vi "Configure.vi"(8 "error in (no error)":errorcluster, 10 "Msg in":T1, 11 "FakePressureController in":refnum<class "Ztec4611.lvclass">) -> (0 "error out":errorcluster, 1 "new command":string, 2 "Msg out":T1, 3 "FakePressureController out":refnum<class "Ztec4611.lvclass">)   [LabVIEW 2011, in "Ztec4611.lvclass"]
uses:
  Ztec4611.lvclass
  DriverMsg.ctl
  Ztec4611.lvclass/Ztec4611.ctl
  impedance_Enum_TypDEf.ctl
  OnOffTypeDef.ctl
  coupling_Enum_TypDef.ctl
  TriggerSource_TypDef.ctl
  positive_negatice2_typDef.ctl
  mode_TypDef.ctl
  BaseDriver/BaseDriver.lvclass
panel:
  out "Command":string
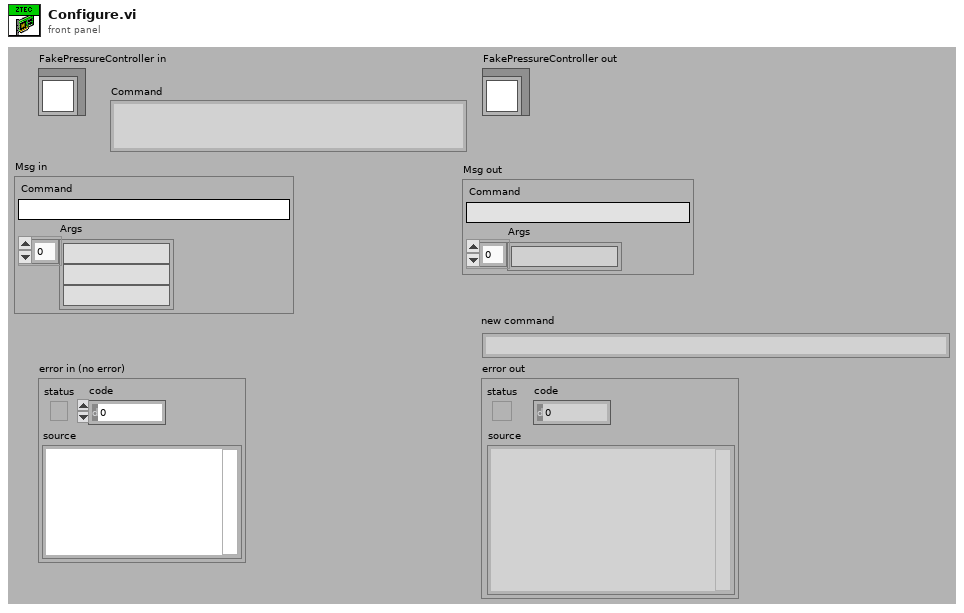
[diagram p1: front panel]
types:
  T1 = typedef "DriverMsg.ctl" = cluster{"Command":string, "Args":string[]}
  T2 = typedef "impedance_Enum_TypDEf.ctl" = enum16{"1 mega ohm", "<NA>", "50 ohms"}
  T3 = typedef "OnOffTypeDef.ctl" = enum16{"off", "on"}
  T4 = typedef "coupling_Enum_TypDef.ctl" = enum16{"AC", "DC", "Ground"}
  T5 = typedef "TriggerSource_TypDef.ctl" = enum16{"Channel 0", "Channel 1", "External TRIG"}
  T6 = typedef "positive_negatice2_typDef.ctl" = enum16{"Positive", "Negative"}
  T7 = typedef "mode_TypDef.ctl" = enum32{"Immediate", "Analog Edge", "Analog Window", "Analog Hysteresis", "Video", "Digital Edge"}
  T8 = typedef "Ztec4611.lvclass/settings_TypDef.ctl" = cluster{"resourcename":string, "timeout":T9, "LocalSavingPath":path, "Save":T3, "probeattenuation":cluster{"Channel0":T9, "Channel1":T9, "Channel2":T9, "Channel3":T9, "Channel4":T9, "Channel5":T9, "Channel6":T9, "Channel7":T9}, "channelenabled":T10, "coupling":cluster{"Channel0":T4, "Channel1":T4, "Channel2":T4, "Channel3":T4, "Channel4":T4, "Channel5":T4, "Channel6":T4, "Channel7":T4}, "impedance":cluster{"Channel0":T2, "Channel1":T2, "Channel2":T2, "Channel3":T2, "Channel4":T2, "Channel5":T2, "Channel6":T2, "Channel7":T2}, "Trigger":cluster{"Slope":T6, "AnalogSource":T5, "Low Level":dbl, "Delay":dbl, "Mode":T7}, "Horizontal":T11, "Names":cluster{"Channel0":string, "Channel1":string, "Channel2":string, "Channel3":string, "Channel4":string, "Channel5":string, "Channel6":string, "Channel7":string}, "verticalrange":cluster{"Channel0":T9, "Channel1":T9, "Channel2":T9, "Channel3":T9, "Channel4":T9, "Channel5":T9, "Channel6":T9, "Channel7":T9}, "offset":cluster{"Channel0":T9, "Channel1":T9, "Channel2":T9, "Channel3":T9, "Channel4":T9, "Channel5":T9, "Channel6":T9, "Channel7":T9}, "Number of channels":dbl, "Method":T12, "LinkedChannel":T14}
  T9 = typedef "numericVariable_TypeDef.ctl" = cluster{"Value":dbl, "Min":dbl, "Max":dbl, "StepSize":dbl, "Tolerance":dbl, "valueactual":dbl}
  T10 = typedef "channelenabled_TypDef.ctl" = cluster{"Channel0":T3, "Channel1":T3, "Channel2":T3, "Channel3":T3, "Channel4":T3, "Channel5":T3, "Channel6":T3, "Channel7":T3}
  T11 = typedef "horizontal_TypDef.ctl" = cluster{"min sample rate":dbl, "min record length":i32, "actual record length":i32, "actual sample rate":dbl, "Enforce Realtime":T3}
  T12 = typedef "methodCluster_TypDEf.ctl" = cluster{"Analysis1":T13, "Analysis2":T13, "Analysis3":T13, "Analysis4":T13, "Analysis5":T13, "Analysis6":T13, "Analysis7":T13, "Analysis8":T13, "Analysis9":T13, "Analysis10":T13}
  T13 = typedef "method_TypDef.ctl" = enum16{"n/a", "max", "min", "energy"}
  T14 = typedef "LinkedChannelsCluster_TypDef.ctl" = cluster{"Analysis1":T15, "Analysis2":T15, "Analysis3":T15, "Analysis4":T15, "Analysis5":T15, "Analysis6":T15, "Analysis7":T15, "Analysis8":T15, "Analysis9":T15, "Analysis10":T15}
  T15 = typedef "channels_TypDef.ctl" = enum16{"Channel0", "Channel1", "Channel2", "Channel3", "Channel4", "Channel5", "Channel6", "Channel7", "n/a"}
  T16 = cluster{"Channel0":T2, "Channel1":T2, "Channel2":T2, "Channel3":T2, "Channel4":T2, "Channel5":T2, "Channel6":T2, "Channel7":T2}
  T17 = cluster{"Channel0":T4, "Channel1":T4, "Channel2":T4, "Channel3":T4, "Channel4":T4, "Channel5":T4, "Channel6":T4, "Channel7":T4}
  T18 = cluster{"Channel0":T9, "Channel1":T9, "Channel2":T9, "Channel3":T9, "Channel4":T9, "Channel5":T9, "Channel6":T9, "Channel7":T9}
  T19 = cluster{"Channel0":string, "Channel1":string, "Channel2":string, "Channel3":string, "Channel4":string, "Channel5":string, "Channel6":string, "Channel7":string}
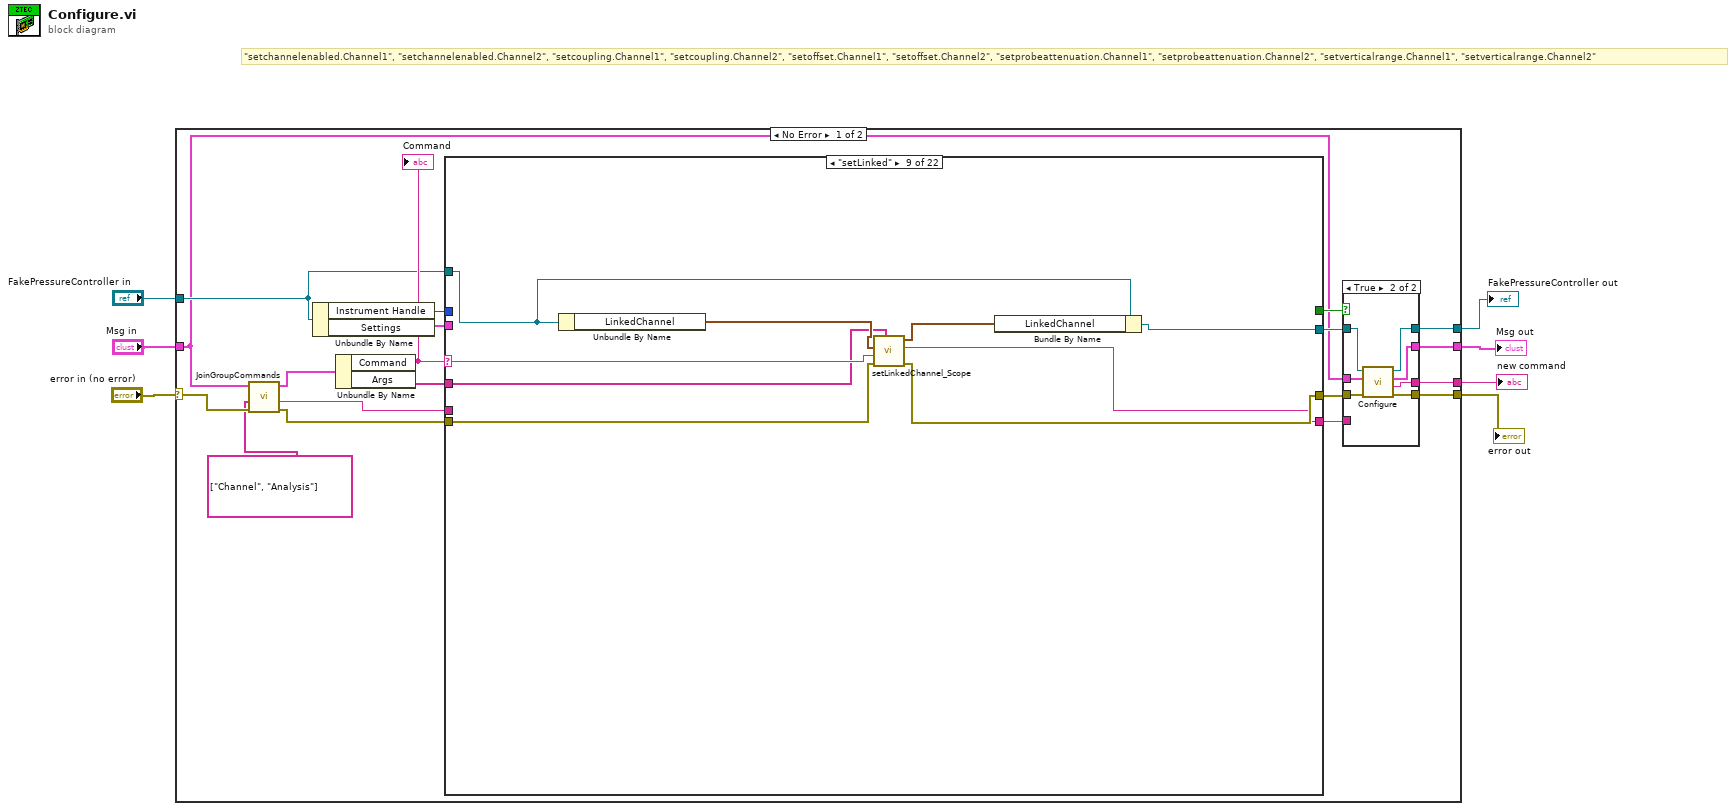
[diagram p0: block diagram]
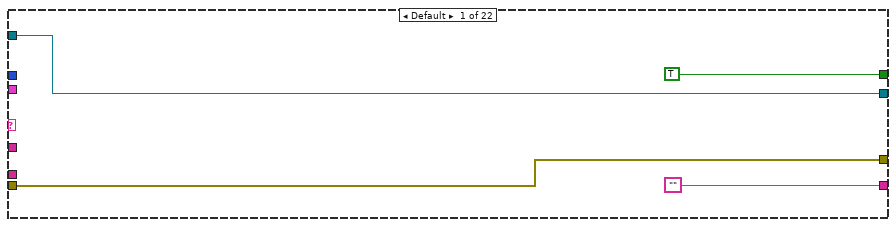
[diagram p3: hidden frame]
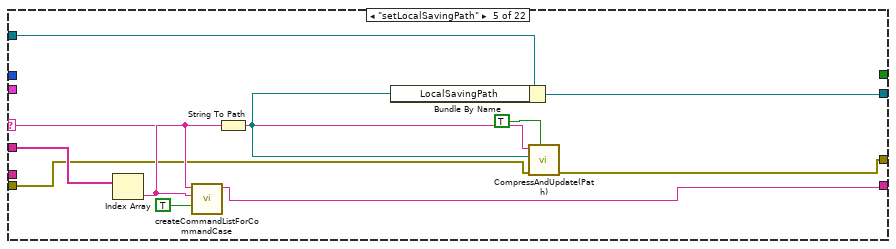
[diagram p7: hidden frame]
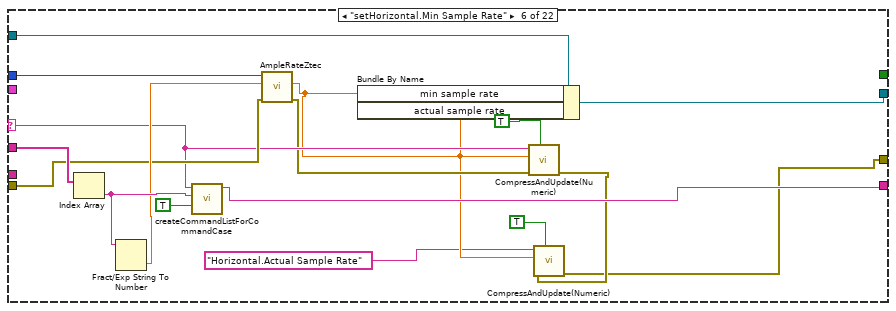
[diagram p8: hidden frame]
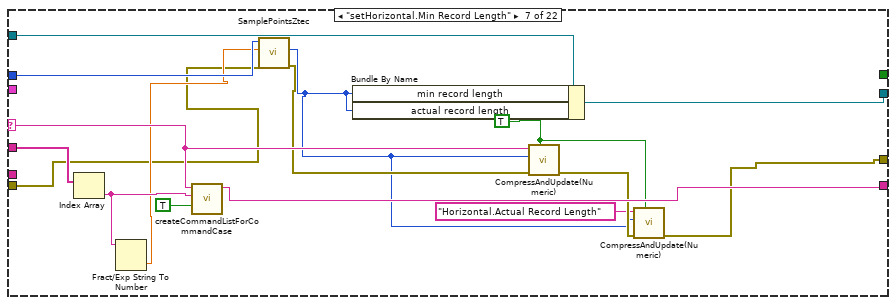
[diagram p9: hidden frame]
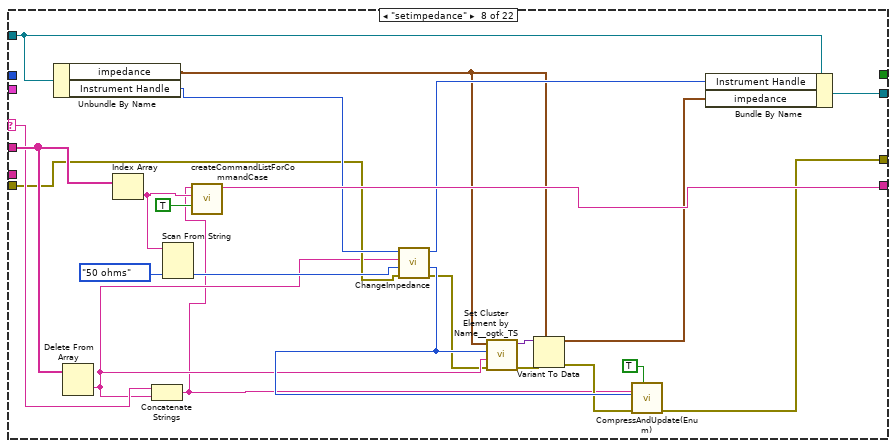
[diagram p10: hidden frame]
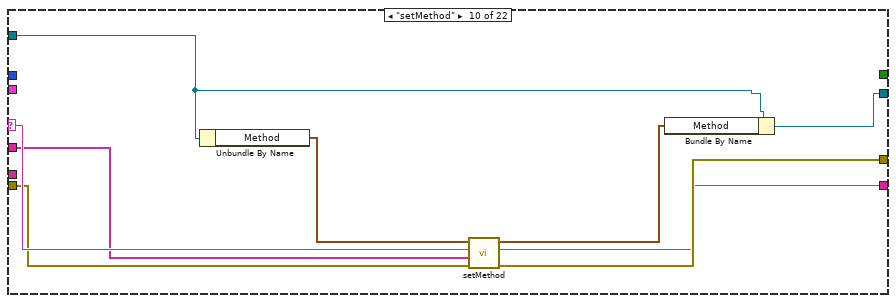
[diagram p11: hidden frame]
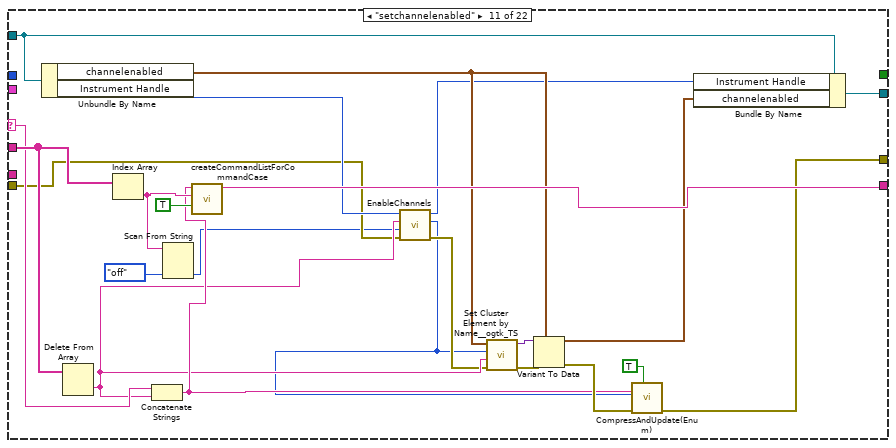
[diagram p12: hidden frame]
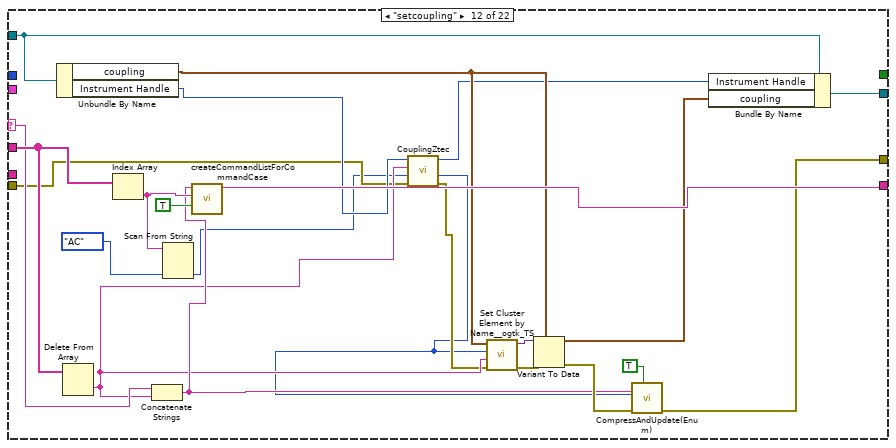
[diagram p13: hidden frame]
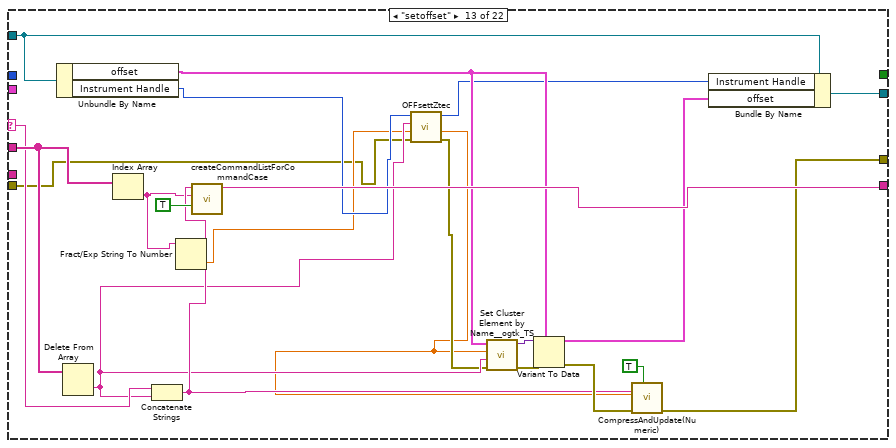
[diagram p14: hidden frame]
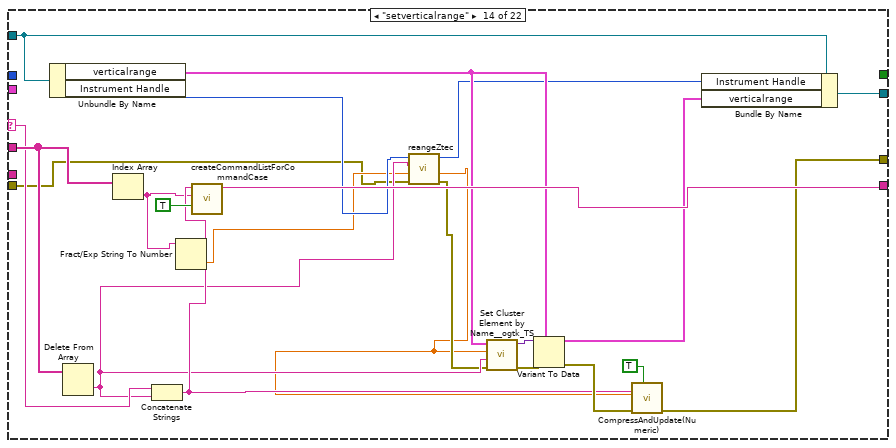
[diagram p15: hidden frame]
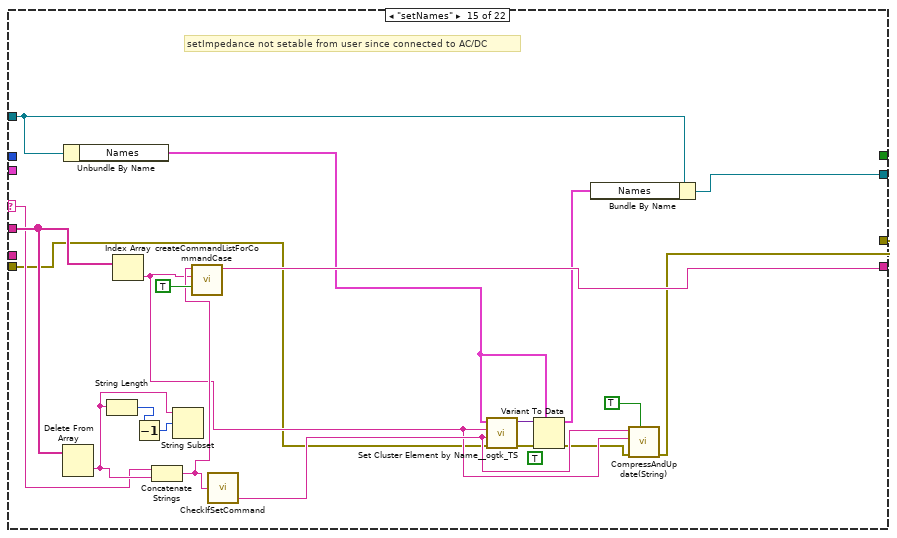
[diagram p16: hidden frame]
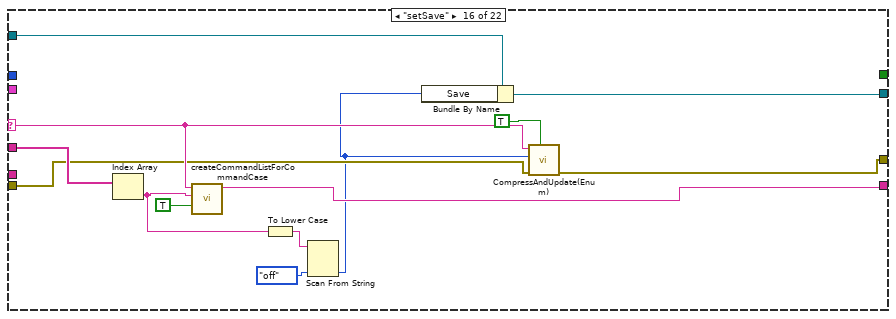
[diagram p17: hidden frame]
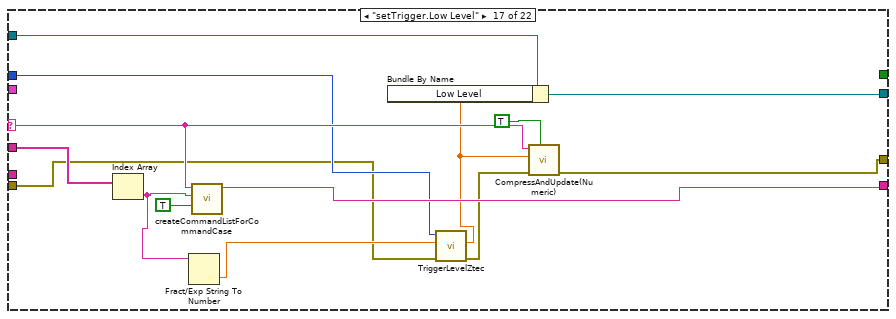
[diagram p18: hidden frame]
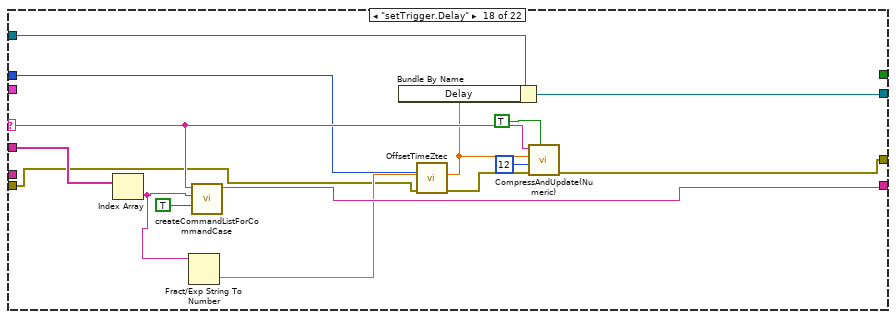
[diagram p19: hidden frame]
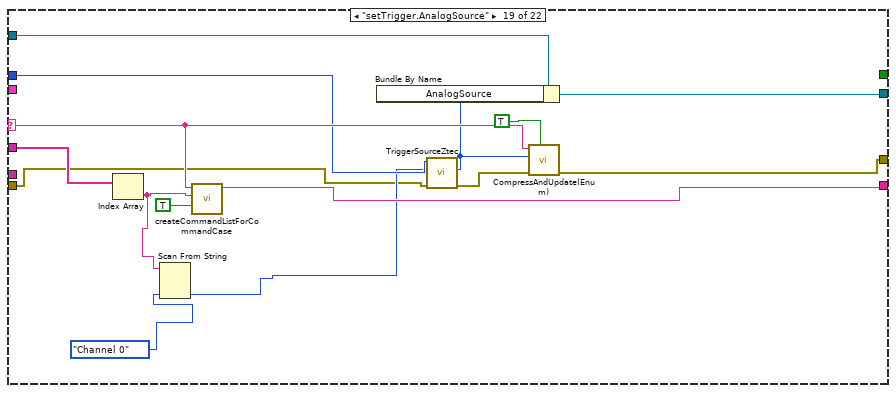
[diagram p20: hidden frame]
diagram:
  # "\"setchannelenabled.Channel1\", \"setchannelenabled.Channel2\", \"setcoupling.Channel1\", \"setcoupling.Channel2\", \"setoffset.Channel1\", \"setoffset.Channel2\", \"setprobeattenuation.Channel1\", \"setprobeattenuation.Channel2\", \"setverticalrange.Channel1\", \"setverticalrange.Channel2\""
  n1 = case shown="No Error" "error in (no error)" {
    selector: "error in (no error)" -> [w13 w356]
    tunnel: "FakePressureController in" -> [w17 w354]
    tunnel: [w25 w354] -> w4
    tunnel: [w23 w356] -> w1
    tunnel: "Msg in" -> [w10 w355]
    tunnel: [w21 w355] -> w3
    tunnel: [w19 _] -> w2
    frame No Error {
      n2 = call "JoinGroupCommands.vi"("error in (no error)"=w13, "Seperator"=string[] ["Channel", "Analysis"], "Msg in"=w10) -> ("error out"=w12:errorcluster, "Seperator out"=w9:string, "Msg out"=w11:T1)  [unwired: 6 in]
      n3 = Unbundle By Name(w17) -> ("Instrument Handle"=w16:i32, "Settings"=w15:T8)
      n4 = Unbundle By Name(w11) -> ("Command"=w18:string, "Args"=w14:string[])
      "Command" <- w18
      n5 = case shown="\"setLinked\"" w18 {
        selector: w18 -> [_ _ _ _ w53 w65 w85 w104 w116 w128 w146 w169 w192 w214 w231 w251 w265 w280 w295 w310 w338 w349]
        tunnel: w12 -> [w40 w43 w45 w46 w50 w66 w82 w99 w119 w126 w136 w161 w181 w203 w225 w249 w257 w273 w287 w304 w333 w347]
        tunnel: w14 -> [_ _ _ _ w56 w73 w89 w108 w115 w127 w150 w173 w196 w218 w236 w253 w267 w282 w297 w312 w340 w351]
        tunnel: w17 -> [w41 w42 w44 w47 w58 w75 w91 w111 w121 w130 w152 w175 w197 w219 w239 w255 w269 w284 w299 w314 w342 w353]
        tunnel: [w41 w42 w44 w47 w48 w70 w87 w112 w120 w129 w153 w176 w198 w220 w240 w247 w262 w277 w292 w307 w335 w345] -> w26
        tunnel: ["" ("Complete") _ _ _ w54 w72 w88 w113 w117 w124 w154 w177 w199 w221 w241 w252 w266 w281 w296 w311 w339 w350] -> w20
        tunnel: [w40 w43 w45 w46 w49 w59 w79 w93 w118 w125 w142 w165 w188 w210 w224 w248 w263 w278 w293 w308 w336 w346] -> w24
        tunnel: [TRUE _ _ _ _ _ _ _ _ _ _ _ _ _ _ _ _ _ _ _ _ _] -> w22
        tunnel: w16 -> [_ _ _ _ _ w69 w84 _ _ _ _ _ _ _ _ _ w259 w275 w290 w305 w332 _]
        tunnel: w15 -> [_ _ _ _ _ _ _ _ _ _ _ _ _ _ _ _ _ _ _ _ _ _]
        tunnel: w9 -> [_ _ _ _ _ _ _ _ _ _ _ _ _ _ _ _ _ _ _ _ _ _]
        frame Default {
        }
        frame "setprobeattenuation" {
        }
        frame "setHorizontal.Enforce Realtime" {
        }
        frame "Abort" {
        }
        frame "setLocalSavingPath" {
          n6 = Index Array(array=w56) -> (element=w55:string)  [unwired: 1 in]
          n7 = call "createCommandListForCommandCase.vi"("immediate Check (only once)"=TRUE, "setvalue"=w55, "command"=w53) -> ("new commands"=w54:string)  [unwired: 8 in]
          n8 = String To Path(string=w55) -> (path=w52:path)
          n9 = Bundle By Name(cluster=w58, "LocalSavingPath"=w52) -> (w48:refnum<class "Ztec4611.lvclass">)
          n10 = call "CompressAndUpdate(Path).vi"("force CVT update (false)"=TRUE, "error in"=w50, "Path"=w52, "command or variable name"=w53) -> ("error out"=w49:errorcluster)  [unwired: 7 in]
        }
        frame "setHorizontal.Min Sample Rate" {
          n11 = Index Array(array=w73) -> (element=w68:string)  [unwired: 1 in]
          n12 = Fract/Exp String To Number(string=w68) -> (number=w67:dbl)  [unwired: 3 in, 1 out]
          n13 = call "createCommandListForCommandCase.vi"("immediate Check (only once)"=TRUE, "setvalue"=w68, "command"=w65) -> ("new commands"=w72:string)  [unwired: 8 in]
          n14 = call "AmpleRateZtec.vi"("error in (no error)"=w66, "NewVal"=w67, "Instrument Handle"=w69) -> ("error out"=w64:errorcluster, "Sample Rate 2"=w62:dbl)  [unwired: 6 in, 1 out]
          n15 = Bundle By Name(cluster=w75, "min sample rate"=w62, "actual sample rate"=w62) -> (w70:refnum<class "Ztec4611.lvclass">)
          n16 = call "CompressAndUpdate(Numeric).vi"("force CVT update (false)"=TRUE, "error in"=w64, "Numeric"=w62, "command or variable name"=w65) -> ("error out"=w60:errorcluster)  [unwired: 7 in]
          n17 = call "CompressAndUpdate(Numeric).vi"("force CVT update (false)"=TRUE, "error in"=w60, "Numeric"=w62, "command or variable name"="Horizontal.Actual Sample Rate") -> ("error out"=w59:errorcluster)  [unwired: 7 in]
        }
        frame "setHorizontal.Min Record Length" {
          w78 = TRUE ("force CVT update (false)")
          n18 = Index Array(array=w89) -> (element=w86:string)  [unwired: 1 in]
          n19 = Fract/Exp String To Number(string=w86) -> (number=w83:dbl)  [unwired: 3 in, 1 out]
          n20 = call "createCommandListForCommandCase.vi"("immediate Check (only once)"=TRUE, "setvalue"=w86, "command"=w85) -> ("new commands"=w88:string)  [unwired: 8 in]
          n21 = call "SamplePointsZtec.vi"("error in (no error)"=w82, "NewVal"=w83, "Instrument Handle"=w84) -> ("error out"=w81:errorcluster, "Sample Points"=w76:u32)  [unwired: 6 in, 1 out]
          n22 = Bundle By Name(cluster=w91, "min record length"=w76, "actual record length"=w76) -> (w87:refnum<class "Ztec4611.lvclass">)
          n23 = call "CompressAndUpdate(Numeric).vi"("force CVT update (false)"=w78, "error in"=w81, "Numeric"=w76, "command or variable name"=w85) -> ("error out"=w80:errorcluster)  [unwired: 7 in]
          n24 = call "CompressAndUpdate(Numeric).vi"("force CVT update (false)"=w78, "error in"=w80, "Numeric"=w76, "command or variable name"="Horizontal.Actual Record Length") -> ("error out"=w79:errorcluster)  [unwired: 7 in]
        }
        frame "setimpedance" {
          n25 = Unbundle By Name(w111) -> ("impedance"=w98:T16, "Instrument Handle"=w103:i32)
          n26 = Delete From Array(array=w108) -> (deleted portion=w97:string)  [unwired: 2 in, 1 out]
          n27 = Index Array(array=w108) -> (element=w110:string)  [unwired: 1 in]
          n28 = Concatenate Strings(w104, w97) -> (w92:string)
          n29 = Scan From String(input string=w110, default 1=impedance_Enum_TypDEf."50 ohms" ("Impedance2")) -> (output 1=w101:T2)  [unwired: 3 in, 3 out]
          n30 = call "createCommandListForCommandCase.vi"("immediate Check (only once)"=TRUE, "setvalue"=w110, "command"=w92) -> ("new commands"=w113:string)  [unwired: 8 in]
          n31 = call "ChangeImpedance.vi"("error in (no error)"=w99, "Impedance"=w101, "Channel (Channel0)"=w97, "Instrument Handle"=w103) -> ("error out"=w95:errorcluster, "Impedance out"=w100:T2, "Instrument Handle Out"=w102:i32)  [unwired: 4 in, 1 out]
          n32 = call "Set Cluster Element by Name__ogtk_TS.vi"("error in (no error)"=w95, "Element Name (\"\": New Element Data Name)"=w97, "New Element Value"=w100, "Cluster"=w98) -> ("error out"=w96:errorcluster, "VCluster out"=w107:variant)  [unwired: 5 in, 1 out]
          n33 = Variant To Data(error in=w96, type=w98, Variant=w107) -> (data=w106:T16, error out=w94:errorcluster)
          n34 = call "CompressAndUpdate(Enum).vi"("force CVT update (false)"=TRUE, "error in"=w94, "enum variant"=w100, "command or variable name"=w92) -> ("error out"=w93:errorcluster)  [unwired: 7 in]
          n35 = Bundle By Name(cluster=w111, "Instrument Handle"=w102, "impedance"=w106) -> (w112:refnum<class "Ztec4611.lvclass">)
        }
        frame "setLinked" {
          n36 = Unbundle By Name(w121) -> ("LinkedChannel"=w123:T14)
          n37 = call "setLinkedChannel_Scope.vi"("Args"=w115, "error in (no error)"=w119, "String"=w116, "Settings.LinkedChannel in"=w123) -> ("error out"=w118:errorcluster, "new commands"=w117:string, "Settings.LinkedChannel out"=w122:T14)  [unwired: 5 in]
          n38 = Bundle By Name(cluster=w121, "LinkedChannel"=w122) -> (w120:refnum<class "Ztec4611.lvclass">)
        }
        frame "setMethod" {
          n39 = Unbundle By Name(w130) -> ("Method"=w132:T12)
          n40 = call "setMethod.vi"("error in (no error)"=w126, "Args"=w127, "String"=w128, "Settings.Method"=w132) -> ("error out"=w125:errorcluster, "new commands"=w124:string, "Settings.Method"=w131:T12)  [unwired: 5 in]
          n41 = Bundle By Name(cluster=w130, "Method"=w131) -> (w129:refnum<class "Ztec4611.lvclass">)
        }
        frame "setchannelenabled" {
          n42 = Unbundle By Name(w152) -> ("channelenabled"=w145:T10, "Instrument Handle"=w139:i32)
          n43 = Delete From Array(array=w150) -> (deleted portion=w137:string)  [unwired: 2 in, 1 out]
          n44 = Index Array(array=w150) -> (element=w151:string)  [unwired: 1 in]
          n45 = Concatenate Strings(w146, w137) -> (w141:string)
          n46 = Scan From String(input string=w151, default 1=OnOffTypeDef."off" ("Settings.Trigger")) -> (output 1=w135:T3)  [unwired: 3 in, 3 out]
          n47 = call "createCommandListForCommandCase.vi"("immediate Check (only once)"=TRUE, "setvalue"=w151, "command"=w141) -> ("new commands"=w154:string)  [unwired: 8 in]
          n48 = call "EnableChannels.vi"("error in (no error)"=w136, "enable"=w135, "Channel (Channel0) in"=w137, "Instrument Handle In"=w139) -> ("error out"=w134:errorcluster, "State out"=w133:T3, "Instrument Handle Out"=w138:i32)  [unwired: 5 in]
          n49 = call "Set Cluster Element by Name__ogtk_TS.vi"("error in (no error)"=w134, "Element Name (\"\": New Element Data Name)"=w137, "New Element Value"=w133, "Cluster"=w145) -> ("error out"=w144:errorcluster, "VCluster out"=w149:variant)  [unwired: 5 in, 1 out]
          n50 = Variant To Data(error in=w144, type=w145, Variant=w149) -> (data=w148:T10, error out=w143:errorcluster)
          n51 = call "CompressAndUpdate(Enum).vi"("force CVT update (false)"=TRUE, "error in"=w143, "enum variant"=w133, "command or variable name"=w141) -> ("error out"=w142:errorcluster)  [unwired: 7 in]
          n52 = Bundle By Name(cluster=w152, "Instrument Handle"=w138, "channelenabled"=w148) -> (w153:refnum<class "Ztec4611.lvclass">)
        }
        frame "setcoupling" {
          n53 = Unbundle By Name(w175) -> ("coupling"=w168:T17, "Instrument Handle"=w163:i32)
          n54 = Delete From Array(array=w173) -> (deleted portion=w162:string)  [unwired: 2 in, 1 out]
          n55 = Index Array(array=w173) -> (element=w174:string)  [unwired: 1 in]
          n56 = Concatenate Strings(w169, w162) -> (w164:string)
          n57 = Scan From String(input string=w174, default 1=coupling_Enum_TypDef."AC" ("coupling")) -> (output 1=w158:T4)  [unwired: 3 in, 3 out]
          n58 = call "createCommandListForCommandCase.vi"("immediate Check (only once)"=TRUE, "setvalue"=w174, "command"=w164) -> ("new commands"=w177:string)  [unwired: 8 in]
          n59 = call "CouplingZtec.vi"("error in (no error)"=w161, "coupling"=w158, "Channel (Channel0)"=w162, "Instrument Handle"=w163) -> ("error out"=w160:errorcluster, "coupling"=w157:T4, "Instrument Handle Out"=w159:i32)  [unwired: 4 in, 1 out]
          n60 = call "Set Cluster Element by Name__ogtk_TS.vi"("error in (no error)"=w160, "Element Name (\"\": New Element Data Name)"=w162, "New Element Value"=w157, "Cluster"=w168) -> ("error out"=w167:errorcluster, "VCluster out"=w172:variant)  [unwired: 5 in, 1 out]
          n61 = Variant To Data(error in=w167, type=w168, Variant=w172) -> (data=w171:T17, error out=w166:errorcluster)
          n62 = call "CompressAndUpdate(Enum).vi"("force CVT update (false)"=TRUE, "error in"=w166, "enum variant"=w157, "command or variable name"=w164) -> ("error out"=w165:errorcluster)  [unwired: 7 in]
          n63 = Bundle By Name(cluster=w175, "Instrument Handle"=w159, "coupling"=w171) -> (w176:refnum<class "Ztec4611.lvclass">)
        }
        frame "setoffset" {
          n64 = Unbundle By Name(w197) -> ("offset"=w191:T18, "Instrument Handle"=w186:i32)
          n65 = Delete From Array(array=w196) -> (deleted portion=w184:string)  [unwired: 2 in, 1 out]
          n66 = Index Array(array=w196) -> (element=w183:string)  [unwired: 1 in]
          n67 = Concatenate Strings(w192, w184) -> (w187:string)
          n68 = Fract/Exp String To Number(string=w183) -> (number=w182:dbl)  [unwired: 3 in, 1 out]
          n69 = call "createCommandListForCommandCase.vi"("immediate Check (only once)"=TRUE, "setvalue"=w183, "command"=w187) -> ("new commands"=w199:string)  [unwired: 8 in]
          n70 = call "OFFsettZtec.vi"("error in (no error)"=w181, "offset"=w182, "Channel (Channel0)"=w184, "Instrument Handle"=w186) -> ("error out"=w180:errorcluster, "Offset out"=w179:dbl, "Instrument Handle Out"=w185:i32)  [unwired: 4 in, 1 out]
          n71 = call "Set Cluster Element by Name__ogtk_TS.vi"("error in (no error)"=w180, "Element Name (\"\": New Element Data Name)"=w184, "New Element Value"=w179, "Cluster"=w191) -> ("error out"=w190:errorcluster, "VCluster out"=w195:variant)  [unwired: 5 in, 1 out]
          n72 = Variant To Data(error in=w190, type=w191, Variant=w195) -> (data=w194:T18, error out=w189:errorcluster)
          n73 = call "CompressAndUpdate(Numeric).vi"("force CVT update (false)"=TRUE, "error in"=w189, "Numeric"=w179, "command or variable name"=w187) -> ("error out"=w188:errorcluster)  [unwired: 7 in]
          n74 = Bundle By Name(cluster=w197, "Instrument Handle"=w185, "offset"=w194) -> (w198:refnum<class "Ztec4611.lvclass">)
        }
        frame "setverticalrange" {
          n75 = Unbundle By Name(w219) -> ("verticalrange"=w213:T18, "Instrument Handle"=w207:i32)
          n76 = Delete From Array(array=w218) -> (deleted portion=w205:string)  [unwired: 2 in, 1 out]
          n77 = Index Array(array=w218) -> (element=w208:string)  [unwired: 1 in]
          n78 = Concatenate Strings(w214, w205) -> (w209:string)
          n79 = Fract/Exp String To Number(string=w208) -> (number=w204:dbl)  [unwired: 3 in, 1 out]
          n80 = call "createCommandListForCommandCase.vi"("immediate Check (only once)"=TRUE, "setvalue"=w208, "command"=w209) -> ("new commands"=w221:string)  [unwired: 8 in]
          n81 = call "reangeZtec.vi"("error in (no error)"=w203, "NewVal"=w204, "Channel (Channel0)"=w205, "Instrument Handle"=w207) -> ("error out"=w202:errorcluster, "Range out"=w201:dbl, "Instrument Handle Out"=w206:i32)  [unwired: 4 in, 1 out]
          n82 = call "Set Cluster Element by Name__ogtk_TS.vi"("error in (no error)"=w202, "Element Name (\"\": New Element Data Name)"=w205, "New Element Value"=w201, "Cluster"=w213) -> ("error out"=w212:errorcluster, "VCluster out"=w217:variant)  [unwired: 5 in, 1 out]
          n83 = Variant To Data(error in=w212, type=w213, Variant=w217) -> (data=w216:T18, error out=w211:errorcluster)
          n84 = call "CompressAndUpdate(Numeric).vi"("force CVT update (false)"=TRUE, "error in"=w211, "Numeric"=w201, "command or variable name"=w209) -> ("error out"=w210:errorcluster)  [unwired: 7 in]
          n85 = Bundle By Name(cluster=w219, "Instrument Handle"=w206, "verticalrange"=w216) -> (w220:refnum<class "Ztec4611.lvclass">)
        }
        frame "setNames" {
          (unwired) TRUE ("force CVT update (false)")
          # "setImpedance not setable from user since connected to AC/DC"
          n86 = Delete From Array(array=w236) -> (deleted portion=w235:string)  [unwired: 2 in, 1 out]
          n87 = Unbundle By Name(w239) -> ("Names"=w233:T19)
          n88 = String Length(string=w235) -> (length=w238:i32)
          n89 = Index Array(array=w236) -> (element=w228:string)  [unwired: 1 in]
          n90 = Decrement(x=w238) -> (x-1=w237:i32)
          n91 = Concatenate Strings(w231, w235) -> (w230:string)
          n92 = String Subset(string=w235, offset (0)=w237) -> ()  [unwired: 1 in, 1 out]
          n93 = call "createCommandListForCommandCase.vi"("immediate Check (only once)"=TRUE, "setvalue"=w228, "command"=w230) -> ("new commands"=w241:string)  [unwired: 8 in]
          n94 = call "CheckIfSetCommand.vi"("Command"=w230) -> ("variable"=w229:string)  [unwired: 2 out]
          n95 = call "Set Cluster Element by Name__ogtk_TS.vi"("error in (no error)"=w225, "Element Name (\"\": New Element Data Name)"=w229, "New Element Value"=w228, "Cluster"=w233) -> ("error out"=w226:errorcluster, "VCluster out"=w234:variant)  [unwired: 5 in, 1 out]
          n96 = Variant To Data(error in=w226, type=w233, Variant=w234) -> (data=w232:T19, error out=w227:errorcluster)
          n97 = Bundle By Name(cluster=w239, "Names"=w232) -> (w240:refnum<class "Ztec4611.lvclass">)
          n98 = call "CompressAndUpdate(String).vi"("force CVT update (false)"=TRUE, "error in"=w227, "String"=w228, "command or variable name"=w229) -> ("error out"=w224:errorcluster)  [unwired: 7 in]
        }
        frame "setSave" {
          n99 = Index Array(array=w253) -> (element=w244:string)  [unwired: 1 in]
          n100 = call "createCommandListForCommandCase.vi"("immediate Check (only once)"=TRUE, "setvalue"=w244, "command"=w251) -> ("new commands"=w252:string)  [unwired: 8 in]
          n101 = To Lower Case(string=w244) -> (all lower case string=w246:string)
          n102 = Scan From String(input string=w246, default 1=OnOffTypeDef."off" ("Settings.Trigger")) -> (output 1=w243:T3)  [unwired: 3 in, 3 out]
          n103 = Bundle By Name(cluster=w255, "Save"=w243) -> (w247:refnum<class "Ztec4611.lvclass">)
          n104 = call "CompressAndUpdate(Enum).vi"("force CVT update (false)"=TRUE, "error in"=w249, "enum variant"=w243, "command or variable name"=w251) -> ("error out"=w248:errorcluster)  [unwired: 7 in]
        }
        frame "setTrigger.Low Level" {
          n105 = Index Array(array=w267) -> (element=w261:string)  [unwired: 1 in]
          n106 = Fract/Exp String To Number(string=w261) -> (number=w260:dbl)  [unwired: 3 in, 1 out]
          n107 = call "createCommandListForCommandCase.vi"("immediate Check (only once)"=TRUE, "setvalue"=w261, "command"=w265) -> ("new commands"=w266:string)  [unwired: 8 in]
          n108 = call "TriggerLevelZtec.vi"("error in (no error)"=w257, "NewVal"=w260, "Instrument Handle"=w259) -> ("error out"=w256:errorcluster, "Level 2"=w258:dbl)  [unwired: 6 in, 1 out]
          n109 = Bundle By Name(cluster=w269, "Low Level"=w258) -> (w262:refnum<class "Ztec4611.lvclass">)
          n110 = call "CompressAndUpdate(Numeric).vi"("force CVT update (false)"=TRUE, "error in"=w256, "Numeric"=w258, "command or variable name"=w265) -> ("error out"=w263:errorcluster)  [unwired: 7 in]
        }
        frame "setTrigger.Delay" {
          n111 = Index Array(array=w282) -> (element=w276:string)  [unwired: 1 in]
          n112 = Fract/Exp String To Number(string=w276) -> (number=w274:dbl)  [unwired: 3 in, 1 out]
          n113 = call "createCommandListForCommandCase.vi"("immediate Check (only once)"=TRUE, "setvalue"=w276, "command"=w280) -> ("new commands"=w281:string)  [unwired: 8 in]
          n114 = call "OffsetTimeZtec.vi"("error in (no error)"=w273, "NewVal"=w274, "Instrument Handle"=w275) -> ("error out"=w272:errorcluster, "Offset Time"=w271:dbl)  [unwired: 6 in, 1 out]
          n115 = Bundle By Name(cluster=w284, "Delay"=w271) -> (w277:refnum<class "Ztec4611.lvclass">)
          n116 = call "CompressAndUpdate(Numeric).vi"("force CVT update (false)"=TRUE, "error in"=w272, "precision (6)"=i16 12, "Numeric"=w271, "command or variable name"=w280) -> ("error out"=w278:errorcluster)  [unwired: 6 in]
        }
        frame "setTrigger.AnalogSource" {
          n117 = Index Array(array=w297) -> (element=w291:string)  [unwired: 1 in]
          n118 = Scan From String(input string=w291, default 1=TriggerSource_TypDef."Channel 0" ("Source")) -> (output 1=w289:T5)  [unwired: 3 in, 3 out]
          n119 = call "createCommandListForCommandCase.vi"("immediate Check (only once)"=TRUE, "setvalue"=w291, "command"=w295) -> ("new commands"=w296:string)  [unwired: 8 in]
          n120 = call "TriggerSourceZtec.vi"("error in (no error)"=w287, "Source"=w289, "Instrument Handle"=w290) -> ("error out"=w286:errorcluster, "Source"=w288:T5)  [unwired: 6 in, 1 out]
          n121 = Bundle By Name(cluster=w299, "AnalogSource"=w288) -> (w292:refnum<class "Ztec4611.lvclass">)
          n122 = call "CompressAndUpdate(Enum).vi"("force CVT update (false)"=TRUE, "error in"=w286, "enum variant"=w288, "command or variable name"=w295) -> ("error out"=w293:errorcluster)  [unwired: 7 in]
        }
        frame "setTrigger.Slope" {
          n123 = Index Array(array=w312) -> (element=w306:string)  [unwired: 1 in]
          n124 = Scan From String(input string=w306, default 1=positive_negatice2_typDef."Positive" ("Settings.Trigger.Slope")) -> (output 1=w302:T6)  [unwired: 3 in, 3 out]
          n125 = call "createCommandListForCommandCase.vi"("immediate Check (only once)"=TRUE, "setvalue"=w306, "command"=w310) -> ("new commands"=w311:string)  [unwired: 8 in]
          n126 = call "TriggerSlopeZtec.vi"("error in (no error)"=w304, "Settings.Trigger.Slope"=w302, "Instrument Handle"=w305) -> ("error out"=w303:errorcluster, "Settings.Trigger.Slope"=w300:T6)  [unwired: 6 in, 1 out]
          n127 = Bundle By Name(cluster=w314, "Slope"=w300) -> (w307:refnum<class "Ztec4611.lvclass">)
          n128 = call "CompressAndUpdate(Enum).vi"("force CVT update (false)"=TRUE, "error in"=w303, "enum variant"=w300, "command or variable name"=w310) -> ("error out"=w308:errorcluster)  [unwired: 7 in]
        }
        frame "setTrigger.Mode" {
          w319 = 1 items=["Auto", "Normal"] ("Trigger Mode")
          w323 = 0 items=["Auto", "Normal"] ("Trigger Mode")
          w324 = 1 items=["Auto", "Normal"] ("Trigger Mode")
          w326 = mode_TypDef."Analog Edge" ("Settings.Trigger.Mode")
          n129 = Index Array(array=w340) -> (element=w334:string)  [unwired: 1 in]
          n130 = Scan From String(input string=w334, default 1=w326) -> (output 1=w327:T7)  [unwired: 3 in, 3 out]
          n131 = call "createCommandListForCommandCase.vi"("immediate Check (only once)"=TRUE, "setvalue"=w334, "command"=w338) -> ("new commands"=w339:string)  [unwired: 8 in]
          n132 = Equal?(x=w327, y=w326) -> (x = y?=w325:bool)
          n133 = Select(t=w324, s=w325, f=w323) -> (s? t:f=w322:i32)
          n134 = call "ztscopeM Acquisition Query.vi"("Instrument Handle In"=w332) -> ("Acquire Count"=w329:i32, "Acquire Type"=w330:i32, "Instrument Handle Out"=w331:i32, "Initiate Continuously"=w328:i32)  [unwired: 5 in, 2 out]
          n135 = call "ztscopeM Acquisition.vi"("Trigger Mode"=w322, "Initiate Continuously"=w328, "Acquire Count"=w329, "Acquire Type"=w330, "Instrument Handle In"=w331) -> ("Instrument Handle Out"=w321:i32)  [unwired: 5 in, 1 out]
          n136 = call "ztscopeM Acquisition Query.vi"("Instrument Handle In"=w321) -> ("Trigger Mode"=w320:i32)  [unwired: 5 in, 5 out]
          n137 = Equal?(x=w319, y=w320) -> (x = y?=w318:bool)
          n138 = Select(t=mode_TypDef."Analog Edge" ("Settings.Trigger.Mode"), s=w318, f=mode_TypDef."Immediate" ("Settings.Trigger.Mode")) -> (s? t:f=w315:T7)
          n139 = Bundle By Name(cluster=w342, "Mode"=w315) -> (w335:refnum<class "Ztec4611.lvclass">)
          n140 = call "CompressAndUpdate(Enum).vi"("force CVT update (false)"=TRUE, "error in"=w333, "enum variant"=w315, "command or variable name"=w338) -> ("error out"=w336:errorcluster)  [unwired: 7 in]
        }
        frame "settimeout" {
          n141 = Index Array(array=w351) -> (element=w344:string)  [unwired: 1 in]
          n142 = call "createCommandListForCommandCase.vi"("immediate Check (only once)"=TRUE, "setvalue"=w344, "command"=w349) -> ("new commands"=w350:string)  [unwired: 8 in]
          n143 = Fract/Exp String To Number(string=w344) -> (number=w343:dbl)  [unwired: 3 in, 1 out]
          n144 = Bundle By Name(cluster=w353, "Value"=w343) -> (w345:refnum<class "Ztec4611.lvclass">)
          n145 = call "CompressAndUpdate(Numeric).vi"("force CVT update (false)"=TRUE, "error in"=w347, "Numeric"=w343, "command or variable name"=w349) -> ("error out"=w346:errorcluster)  [unwired: 7 in]
        }
      }
      n146 = case shown="True" w22 {
        tunnel: w26 -> [w28 w37]
        tunnel: [w28 w36] -> w25
        tunnel: [w29 w35] -> w19
        tunnel: w24 -> [w27 w34]
        tunnel: [w27 w33] -> w23
        tunnel: w10 -> [w30 w32]
        tunnel: [w30 w31] -> w21
        tunnel: w20 -> [w29 _]
        frame False {
        }
        frame True {
          n147 = call-parent "Configure.vi"("error in (no error)"=w34, "Msg in"=w32, "BaseDriver in"=w37) -> ("error out"=w33:errorcluster, "new command"=w35:string, "Msg out"=w31:T1, "BaseDriver out"=w36:refnum<class "Ztec4611.lvclass">)  [unwired: 5 in]
        }
      }
    }
    frame Error {
    }
  }
  "error out" <- w1
  "FakePressureController out" <- w4
  "new command" <- w2
  "Msg out" <- w3
